vi "zmqPull.vi"(0 "socket in":refnum<class "zmq_socket.lvclass">, 11 "error in":errorcluster) -> (1 "X":dbl format="%.2f", 2 "Y":dbl format="%.2f", 3 "Z":dbl format="%.2f", 4 "socket out":refnum<class "zmq_socket.lvclass">, 8 "state":T1, 12 "velocity":dbl format="%.2f", 13 "accel.":dbl format="%.2f", 14 "deccel.":dbl format="%.2f", 15 "error out":errorcluster)   [LabVIEW 2020]
uses:
  states.ctl
  <vilib>/addons/zeromq/zmq_socket.lvclass
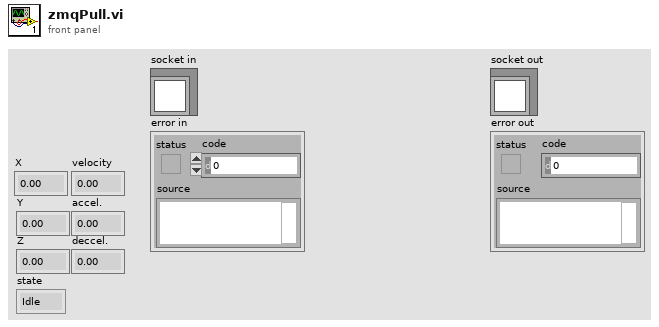
[diagram p1: front panel]
types:
  T1 = typedef "states.ctl" = enum16{"Idle", "Home", "Move", "DisableAxis", "HomePosition", "Stop"}
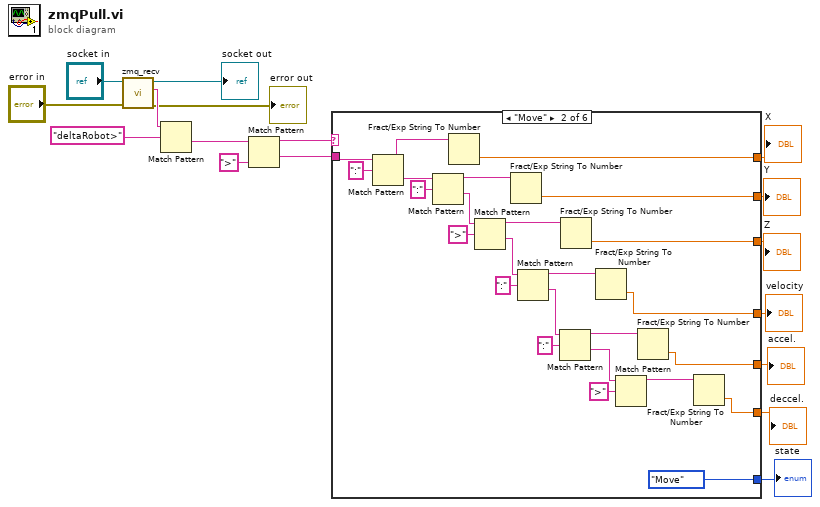
[diagram p0: block diagram]
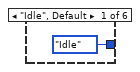
[diagram p2: hidden frame]
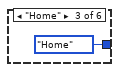
[diagram p3: hidden frame]
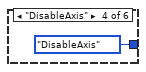
[diagram p4: hidden frame]
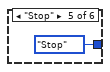
[diagram p5: hidden frame]
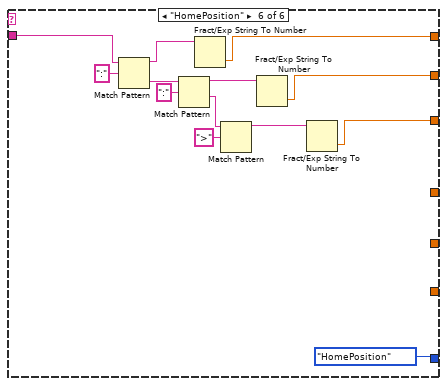
[diagram p6: hidden frame]
diagram:
  n1 = call <vilib>:"zmq_recv.vi"("error in"="error in", "socket in"="socket in") -> ("error out"=→"error out":errorcluster, "data"=w5:string, "socket out"=→"socket out":refnum<class "zmq_socket.lvclass">)  [unwired: 3 in, 2 out]
  n2 = Match Pattern(string=w5, regular expression="deltaRobot>" ("y")) -> (after substring=w16:string)  [unwired: 1 in, 3 out]
  n3 = Match Pattern(string=w16, regular expression=">") -> (before substring=w14:string, after substring=w13:string)  [unwired: 1 in, 2 out]
  n4 = case shown="\"Move\"" w14 {
    tunnel: w13 -> [_ w43 _ _ _ w52]
    tunnel: [_ w40 _ _ _ w50] -> w12
    tunnel: [_ w36 _ _ _ w49] -> w11
    tunnel: [_ w32 _ _ _ w48] -> w10
    tunnel: [_ w28 _ _ _ _] -> w9
    tunnel: [_ w21 _ _ _ _] -> w8
    tunnel: [_ w20 _ _ _ _] -> w7
    tunnel: [states."Idle" states."Move" states."Home" states."DisableAxis" states."Stop" states."HomePosition"] -> w6
    frame "Idle", Default {
    }
    frame "Move" {
      n5 = Match Pattern(string=w43, regular expression=":") -> (before substring=w41:string, after substring=w38:string)  [unwired: 1 in, 2 out]
      n6 = Match Pattern(string=w38, regular expression=":") -> (before substring=w37:string, after substring=w33:string)  [unwired: 1 in, 2 out]
      n7 = Fract/Exp String To Number(string=w41) -> (number=w40:dbl)  [unwired: 3 in, 1 out]
      n8 = Match Pattern(string=w33, regular expression=">") -> (before substring=w34:string, after substring=w29:string)  [unwired: 1 in, 2 out]
      n9 = Fract/Exp String To Number(string=w37) -> (number=w36:dbl)  [unwired: 3 in, 1 out]
      n10 = Match Pattern(string=w29, regular expression=":") -> (before substring=w30:string, after substring=w23:string)  [unwired: 1 in, 2 out]
      n11 = Match Pattern(string=w23, regular expression=":") -> (before substring=w26:string, after substring=w22:string)  [unwired: 1 in, 2 out]
      n12 = Fract/Exp String To Number(string=w34) -> (number=w32:dbl)  [unwired: 3 in, 1 out]
      n13 = Fract/Exp String To Number(string=w30) -> (number=w28:dbl)  [unwired: 3 in, 1 out]
      n14 = Match Pattern(string=w22, regular expression=">") -> (before substring=w24:string)  [unwired: 1 in, 3 out]
      n15 = Fract/Exp String To Number(string=w26) -> (number=w20:dbl)  [unwired: 3 in, 1 out]
      n16 = Fract/Exp String To Number(string=w24) -> (number=w21:dbl)  [unwired: 3 in, 1 out]
    }
    frame "Home" {
    }
    frame "DisableAxis" {
    }
    frame "Stop" {
    }
    frame "HomePosition" {
      n17 = Match Pattern(string=w52, regular expression=":") -> (before substring=w51:string, after substring=w57:string)  [unwired: 1 in, 2 out]
      n18 = Match Pattern(string=w57, regular expression=":") -> (before substring=w56:string, after substring=w53:string)  [unwired: 1 in, 2 out]
      n19 = Fract/Exp String To Number(string=w51) -> (number=w50:dbl)  [unwired: 3 in, 1 out]
      n20 = Match Pattern(string=w53, regular expression=">") -> (before substring=w54:string)  [unwired: 1 in, 3 out]
      n21 = Fract/Exp String To Number(string=w56) -> (number=w49:dbl)  [unwired: 3 in, 1 out]
      n22 = Fract/Exp String To Number(string=w54) -> (number=w48:dbl)  [unwired: 3 in, 1 out]
    }
  }
  "X" <- w12
  "Y" <- w11
  "Z" <- w10
  "velocity" <- w9
  "deccel." <- w8
  "accel." <- w7
  "state" <- w6
